vi "geracao_numero_aleatorio.vi"() -> ()   [LabVIEW 2020]
panel:
  in  "stop":bool
  out "Iteracoes":i32
  out "Numero gerado aleatoriamente":dbl
  in  "Numero escolhido":dbl
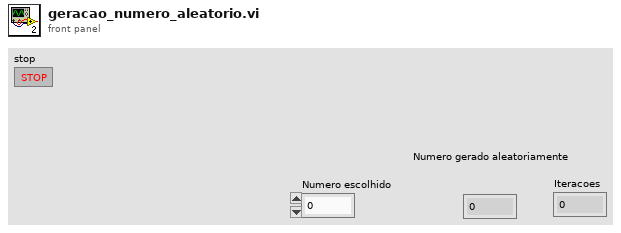
[diagram p1: front panel]
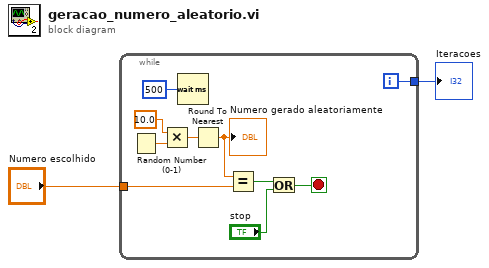
[diagram p0: block diagram]
diagram:
  n1 = while {
    tunnel: "Numero escolhido" -> [w4]
    tunnel: [w3] -> w1
    i -> [w3]
    stop <- w5 stop-if-true
    n2 = Random Number (0-1)() -> (number: 0 to 1=w12:dbl)
    n3 = Multiply(x=10.0, y=w12) -> (x*y=w10:dbl)
    n4 = Wait (ms)(milliseconds to wait=u32 500) -> ()  [unwired: 1 out]
    n5 = Round To Nearest(number=w10) -> (nearest integer value=w9:dbl)
    "Numero gerado aleatoriamente" <- w9
    n6 = Equal?(x=w9, y=w4) -> (x = y?=w8:bool)
    n7 = Or(x=w8, y="stop") -> (x .or. y?=w5:bool)
  }
  "Iteracoes" <- w1
